vi "XLP80_Action_SetCalcAlarms.vi"(8 "err in":errorcluster caption="error") -> (0 "err out":errorcluster caption="error")   [LabVIEW 2021]
uses:
  XLP80_FGlob/1886_FGlob_TDefs_Enum_FGlobItems.ctl
  XLP80_FGlob/1886_FGlob_TDefEnumCANReadItems.ctl
  XLP80_FGlob/XLP80_FGLob_TDefEnumCalcBoolItems.ctl
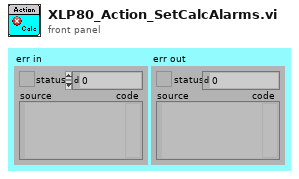
[diagram p1: front panel]
types:
  T1 = typedef "1886_FGlob_TDefs_Enum_FGlobItems.ctl" = enum16{"Put one", "Put all", "Recall one", "Recall all"}
  T2 = typedef "XLP80_FGLob_TDefEnumCalcBoolItems.ctl" = enum8{"Shutdown", "Alarm", "but_NotAus"}
  T3 = typedef "1886_FGlob_TDefEnumCANReadItems.ctl" = enum16{"A03_ETC_a_opCmd1_Start_Stop", "A03_ETC_s_Speed_Actual", "A11_HBV_s_Valve_Act", "A12_SIV_s_Valve_Act", "A13_SOV_s_Valve_Act", "A14_HFM_s_AirMassFlow", "A14_HFM_s_Humidity", "A14_HFM_s_Pressure", "A14_HFM_s_Temperature", "A15_SI_s_Inlet_Pressure", "A15_SI_s_Inlet_Pressure_FM12", "A15_SI_s_Inlet_Temperature", "A16_SI_s_Inlet_Temperature", "A17_SO_s_Outlet_Pressure", "A17_SO_s_Outlet_Pressure_FM12", "A17_SO_s_Outlet_Temperature", "A22_HSI_s_Humidity", "A22_HSI_s_Humidity_FM12", "A23_HSO_s_Humidity", "A56_SO_s_Temperature", "C01_RF_a_FanSpeed", "C02_CP_s_ACTUAL_SPEED_FM2", "C02_CP_a_ENABLE_FM2", "C02_CP_a_RPM", "C04_DI_s_Temperature", "C06_ET_s_CoolLevelStatus", "C07_BAT_s_Board_Temperature", "C07_BAT_s_External_Load_Voltage", "C_07_BAT_s_SoC", "C07_BAT_s_System_Current", "C08_AMB_s_Humidity_Rel", "C08_AMB_s_Pressure", "C08_AMB_s_Temperature", "C24_TRO_s_Temperature_FM23", "C27_RIV_a_Valve_Set_FM2", "C28_RBV_a_Valve_Set_FM2", "C29_TSO_s_Temperature_FM3", "C54_SI_s_Temperature", "C61_SV_a_FanEnable_FM2", "E71_DC4880_s_Current_In_Actual", "E71_DC4880_s_Current_Out_Actual", "E71_DC4880_s_Temperature_1_Act", "E71_DC4880_s_Voltage_Out_Actual", "E71_DC4880_s_Voltage_In_Actual", "E76_HVM_a_Relais_Set", "E75_HVP_a_Relais_Set", "H31_OTV_a_Valve_Set", "H_31_OTV_s_Pressure", "H31_OTV_s_Pressure_FM12", "H_31_OTV_s_Temperature", "H36_GHU_s_Pressure_1", "H36_GHU_s_Pressure_1_FM12", "H37_GHU_s_Temperature_1", "H36_GHU_s_Temperature_FM2", "H38_HSV_a_Valve_Set", "H40_GHU_s_Pressure_2", "H40_GHU_s_Pressure_2_FM12", "H41_GHU_s_Temperature_2", "H42_HRB_s_ARB_Spd", "H43_HDV_a_Dosing_Valve_Set", "H45_WT_s_WaterLevelStatus", "H51_STK_s_CellVolt_highest_2003", "H51_STK_s_CellVolt_lowest_2003", "H51_STK_s_TotalVoltage_2003", "H52_DV_a_Drain_Valve_Stack_Set", "H53_PV_a_Purge_Valve_Stack_Set", "H55_SI_s_Stack_Inlet_Pressure", "H62_HLD_s_H2_Concentration", "H63_HLD_s_H2_Concentration", "H63_HLD_s_concH2_FM2", "S91_SYS_MasterCtrl_State", "S91_SYS_PowerCtrl_State", "S91_SYS_Error_Code", "S91_SYS_Error_Level"}
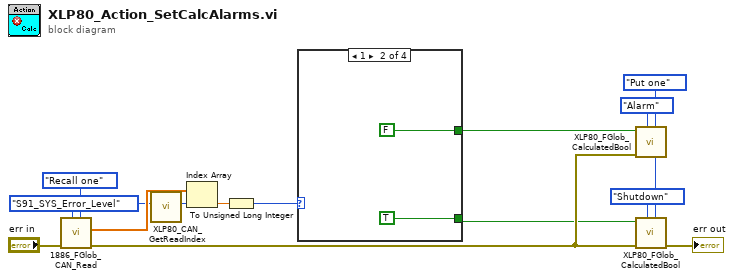
[diagram p0: block diagram]
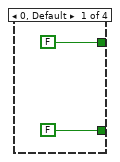
[diagram p2: hidden frame]
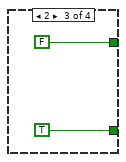
[diagram p3: hidden frame]
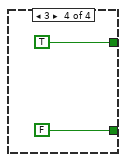
[diagram p4: hidden frame]
diagram:
  w4 = 1886_FGlob_TDefs_Enum_FGlobItems."Put one" ("Function (Recall One)")
  w11 = 1886_FGlob_TDefEnumCANReadItems."S91_SYS_Error_Level" ("CAN Read Items")
  n1 = call "1886_FGlob_CAN_Read.vi"("Function (Recall One)"=1886_FGlob_TDefs_Enum_FGlobItems."Recall one", "CAN Read Items"=w11, "err in"="err in") -> ("err out"=w6:errorcluster, "AI Values OUT"=w13:dbl[])  [unwired: 6 in, 1 out]
  n2 = call "XLP80_CAN_GetReadIndex.vi"("CAN Read Items"=w11) -> ("Index"=w12:i32)  [unwired: 10 in]
  n3 = Index Array(array=w13, index=w12) -> (element=w9:dbl)
  n4 = To Unsigned Long Integer(number=w9) -> (unsigned 32bit integer=w3:u32)
  n5 = case shown="1" w3 {
    tunnel: [FALSE FALSE FALSE TRUE] -> w1
    tunnel: [FALSE TRUE TRUE FALSE] -> w2
    frame 0, Default {
    }
    frame 1 {
    }
    frame 2 {
    }
    frame 3 {
    }
  }
  n6 = call "XLP80_FGlob_CalculatedBool.vi"("Function (Recall One)"=w4, "CalculatedBool_Items"=XLP80_FGLob_TDefEnumCalcBoolItems."Alarm", "err in"=w6, "Calc Value IN"=w1) -> ()  [unwired: 5 in, 3 out]
  n7 = call "XLP80_FGlob_CalculatedBool.vi"("Function (Recall One)"=w4, "CalculatedBool_Items"=XLP80_FGLob_TDefEnumCalcBoolItems."Shutdown", "err in"=w6, "Calc Value IN"=w2) -> ("err out"=→"err out":errorcluster)  [unwired: 5 in, 2 out]
